vi "Replace Outside Items.vi"(0 "Shared directory":path, 5 "OutsideVIs":string[](array[string]), 7 "Dependent VIs":path[](array[path]), 9 "Measurement directory":path, 11 "error in (no error)":errorcluster) -> (15 "error out":errorcluster)   [LabVIEW 2021, in "Multiple Converter.lvlib"]
uses:
  Multiple Converter.lvlib
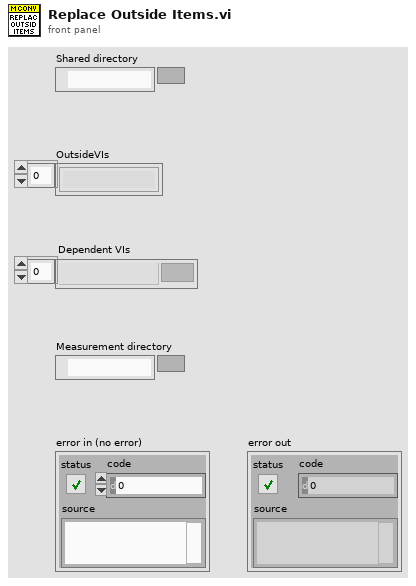
[diagram p1: front panel]
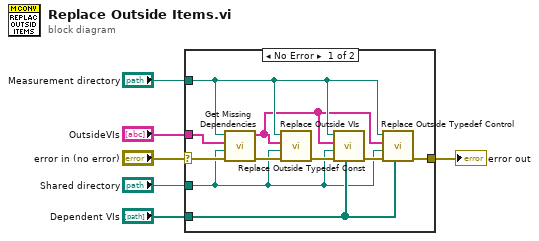
[diagram p0: block diagram]
diagram:
  n1 = case shown="No Error" "error in (no error)" {
    selector: "error in (no error)" -> [w14 w17]
    tunnel: "OutsideVIs" -> [w13 _]
    tunnel: [w12 w17] -> w5
    tunnel: "Measurement directory" -> [w9 _]
    tunnel: "Shared directory" -> [w7 _]
    tunnel: "Dependent VIs" -> [w10 _]
    frame No Error {
      n2 = call "Get Missing Dependencies.vi"("error in (no error)"=w14, "Shared directory"=w7, "OutsideVIs in"=w13, "Measurement directory"=w9) -> ("error out"=w15:errorcluster, "OutsideVIs out"=w8:string[])  [unwired: 6 in]
      n3 = call "Replace Outside VIs.vi"("error in (no error)"=w15, "Shared directory"=w7, "Non-Library VI[]"=w8, "Measurement directory"=w9) -> ("error out"=w16:errorcluster)  [unwired: 7 in]
      n4 = call "Replace Outside Typedef Const.vi"("Dependent VIs"=w10, "error in (no error)"=w16, "Shared directory"=w7, "Non-Library VI[]"=w8, "Measurement Directory"=w9) -> ("error out"=w11:errorcluster)  [unwired: 6 in]
      n5 = call "Replace Outside Typedef Control.vi"("Dependent VIs"=w10, "error in (no error)"=w11, "Shared directory"=w7, "Non-Library VI[]"=w8, "Measurement Directory"=w9) -> ("error out"=w12:errorcluster)  [unwired: 6 in]
    }
    frame Error {
    }
  }
  "error out" <- w5
